vi "listeEmplProjet.vi"(4 "id personnel courant":string, 5 "Suppr/Delete":dbl, 6 "Choix":i16(ring) items=["thibault", "alexis"], 7 "Id projet":string) -> (0 "name":string[](array[string]), 1 "id":string[](array[string]), 2 "size(s)":i32, 3 "String":string)   [LabVIEW 2023]
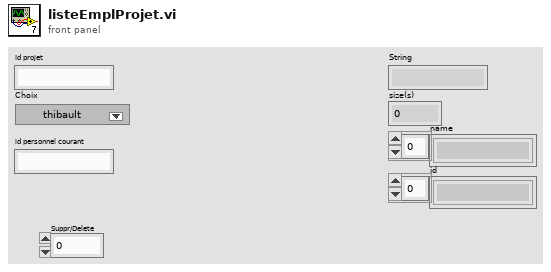
[diagram p1: front panel]
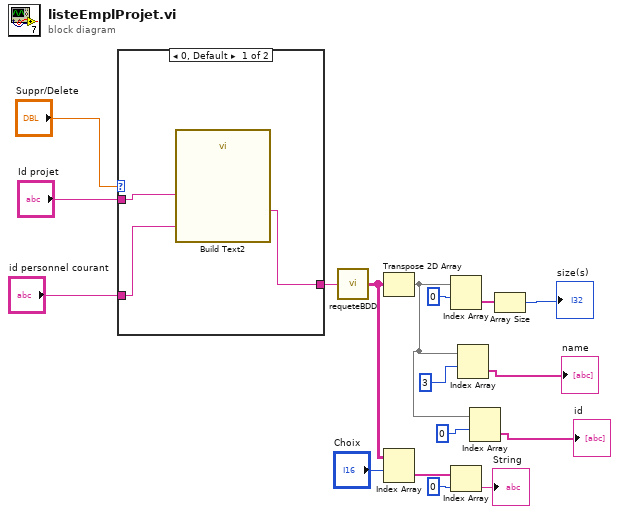
[diagram p0: block diagram]
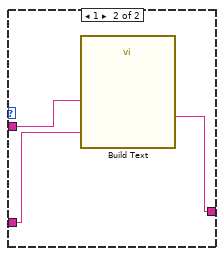
[diagram p2: hidden frame]
diagram:
  n1 = case shown="0, Default" "Suppr/Delete" {
    tunnel: "Id projet" -> [w20 w23]
    tunnel: [w18 w22] -> w16
    tunnel: "id personnel courant" -> [w19 w21]
    frame 0, Default {
      n2 = call "Build Text2"("id"=w20, "id_pers"=w19) -> ("Result"=w18:string)  [unwired: 12 in, 1 out]
    }
    frame 1 {
      n3 = call "Build Text"("id"=w23, "id_pers"=w21) -> ("Result"=w22:string)  [unwired: 12 in, 1 out]
    }
  }
  n4 = call "requeteBDD.vi"("Requête Sql"=w16) -> ("Table Control"=w11:string[][])
  n5 = Transpose 2D Array(2D array=w11) -> (transposed array=w3:string[][])
  n6 = Index Array(array=w11, index (row)="Choix") -> (element=w14:string[])  [unwired: 1 in]
  n7 = Index Array(array=w3, index (row)=0) -> (element=w9:string[])  [unwired: 1 in]
  n8 = Index Array(array=w14, index=0) -> (element=→"String":string)
  n9 = Index Array(array=w3, index (row)=3) -> (element=→"name":string[])  [unwired: 1 in]
  n10 = Index Array(array=w3, index (row)=0) -> (element=→"id":string[])  [unwired: 1 in]
  n11 = Array Size(array=w9) -> (size(s)=→"size(s)":i32)
